vi "AB_RW_Project_Packed_Lib_Info.vi"(7 "action":T1, 8 "error in (no error)":errorcluster, 10 "PackedLib_info in":T2, 11 "Object In":T3) -> (0 "error out":errorcluster, 2 "PackedLib_info out":T2, 3 "Object Out":T3)   [LabVIEW 2020]
uses:
  <resource>/Framework/Providers/API/ItemRef.ctl
  <vilib>/AppBuilder/RW_Project/AB_RW_Project_Packed_Lib_Data.ctl
  <vilib>/AppBuilder/RW_Project/AB_RW_Project_PropBag_Action.ctl
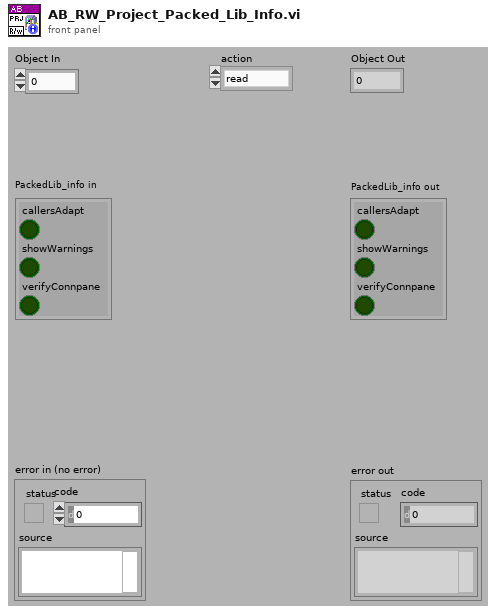
[diagram p1: front panel]
types:
  T1 = typedef "AB_RW_Project_PropBag_Action.ctl" = enum16{"read", "write", "clear", "readPrevious", "writePrevious", "clearPrevious"}
  T2 = typedef "AB_RW_Project_Packed_Lib_Data.ctl" = cluster{"callersAdapt":bool, "showWarnings":bool, "verifyConnpane":bool}
  T3 = typedef "ItemRef.ctl" = u64
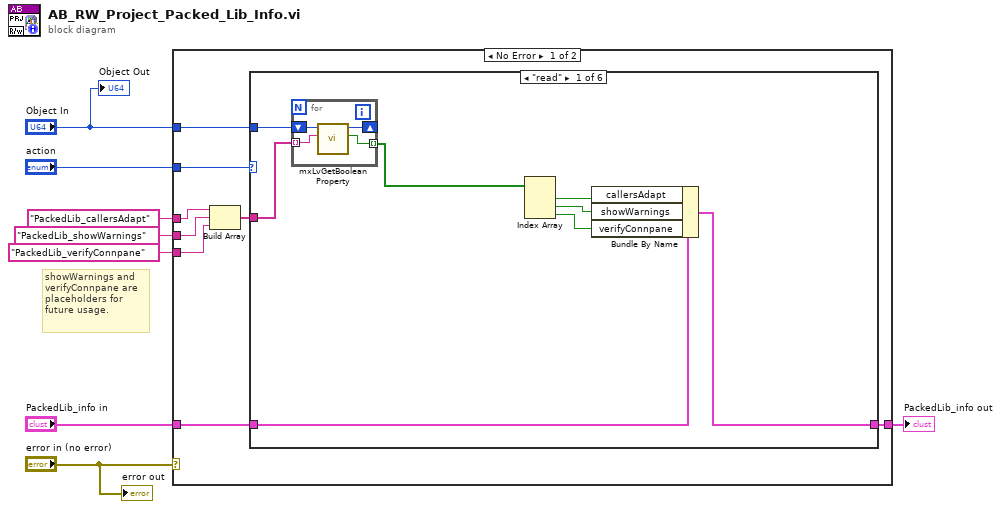
[diagram p0: block diagram]
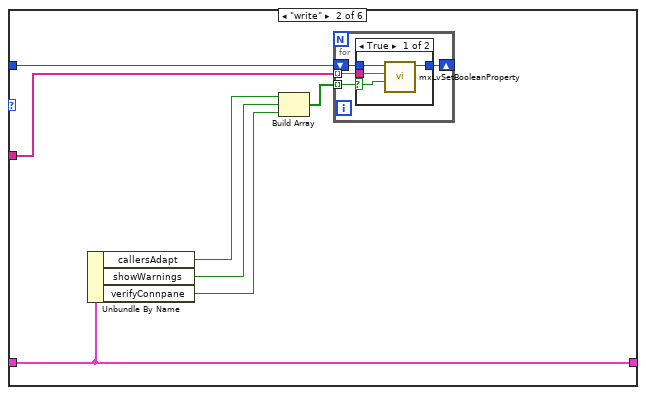
[diagram p2: hidden frame]
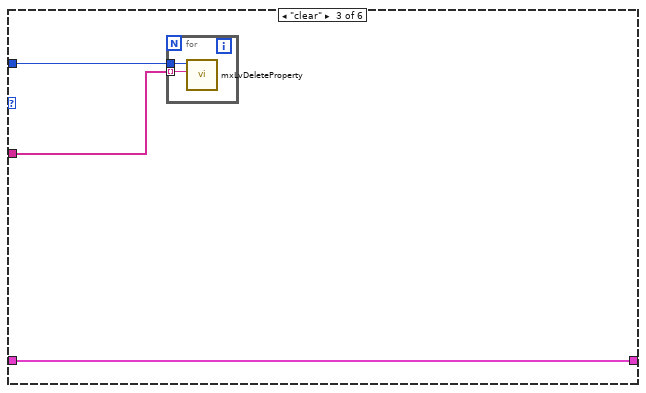
[diagram p4: hidden frame]
diagram:
  # "showWarnings and verifyConnpane are placeholders for future usage."
  n1 = case shown="No Error" "error in (no error)" {
    tunnel: "Object In" -> [w15 _]
    tunnel: [w16 _] -> w6
    tunnel: "PackedLib_info in" -> [w14 _]
    tunnel: "action" -> [w13 _]
    tunnel: "PackedLib_callersAdapt" -> [w12 _]
    tunnel: "PackedLib_showWarnings" ("Tag") -> [w11 _]
    tunnel: "PackedLib_verifyConnpane" ("Tag") -> [w10 _]
    frame No Error {
      n2 = Build Array(w12, w11, w10) -> (w9:string[])
      n3 = case shown="\"read\"" w13 {
        tunnel: [w17 w30 w47 w50 w51 w52] -> w16
        tunnel: w15 -> [w20 w31 w46 _ _ _]
        tunnel: w14 -> [w18 w30 w47 w50 w51 w52]
        tunnel: w9 -> [w19 w29 w45 _ _ _]
        frame "read" {
          n4 = for {
            shift-right: [w27] -> _
            shift-left: w20 -> [w28]
            tunnel: [w26] -> w24 mode=indexing
            tunnel: w19 -> [w25] mode=indexing
            n5 = call <resource>:"mxLvGetBooleanProperty.vi"("Tag"=w25, "Item"=w28) -> ("Value"=w26:bool, "Item"=w27:T3)  [unwired: 7 in, 1 out]
          }
          n6 = Index Array(array=w24) -> (element #1=w23:bool, element #2=w22:bool, element #3=w21:bool)  [unwired: 3 in]
          n7 = Bundle By Name(cluster=w18, "callersAdapt"=w23, "showWarnings"=w22, "verifyConnpane"=w21) -> (w17:T2)
        }
        frame "write" {
          n8 = Unbundle By Name(w30) -> ("callersAdapt"=w35:bool, "showWarnings"=w34:bool, "verifyConnpane"=w33:bool)
          n9 = Build Array(w35, w34, w33) -> (w32:bool[])
          n10 = for {
            tunnel: w32 -> [w38] mode=indexing
            shift-right: [w37] -> _
            shift-left: w31 -> [w39]
            tunnel: w29 -> [w36] mode=indexing
            n11 = case shown="True" w38 {
              selector: w38 -> [w42 _]
              tunnel: w39 -> [w43 w44]
              tunnel: w36 -> [w40 _]
              tunnel: [w41 w44] -> w37
              frame True {
                n12 = call <resource>:"mxLvSetBooleanProperty.vi"("Value (F)"=w42, "Tag"=w40, "Item"=w43) -> ("Item"=w41:T3)  [unwired: 7 in, 1 out]
              }
              frame False {
              }
            }
          }
        }
        frame "clear" {
          n13 = for {
            tunnel: w46 -> [w49]
            tunnel: w45 -> [w48] mode=indexing
            n14 = call <resource>:"mxLvDeleteProperty.vi"("Tag"=w48, "Item"=w49) -> ()  [unwired: 8 in, 2 out]
          }
        }
        frame "readPrevious" {
        }
        frame "writePrevious" {
        }
        frame "clearPrevious" {
        }
      }
    }
    frame Error {
    }
  }
  "PackedLib_info out" <- w6
  "Object Out" <- "Object In"
  "error out" <- "error in (no error)"
